vi "On Click Enumerate Cameras.vi"(8 "error in (no error)":errorcluster, 10 "Value":bool, 11 "App in":refnum<class "App.lvclass">) -> (0 "error out":errorcluster, 3 "App out":refnum<class "App.lvclass">)   [LabVIEW 2020, in "AR Example.lvlib" / "App.lvclass"]
uses:
  App.lvclass
  App.lvclass/App.ctl
  b0e96125-61a1-4303-b342-3e2cae2d3e9f.vi
  917a6586-ad63-4fd0-8dd0-0daf31f14cd0.vi
  <vilib>/Comparison/Equal/Equal Functor/Equal Functor.lvclass
  UI/UI.lvclass
  g_ar_toolkit.capture/CameraStream/CameraStream.lvclass
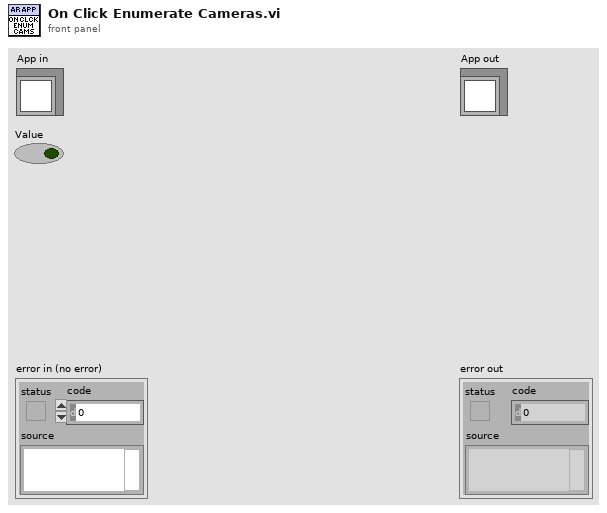
[diagram p1: front panel]
types:
  T1 = enum16{"Set UI Pre Enum", "Enumerate", "Update Lists", "Set UI Post Enum"}
  T2 = enum16{"Set UI Pre Enum", "Enumerate", "Update Lists", "Set UI Post Enum"}[]
  T3 = typedef "g_ar_toolkit.capture.lvlib/CameraStream.lvclass/Device Enumeration.ctl" = cluster{"Name":string, "Streams":set{T4}}
  T4 = typedef "g_ar_toolkit.capture.lvlib/CameraStream.lvclass/Stream Parameters.ctl" = cluster{"Width":u16, "Height":u16, "FPS":u8}
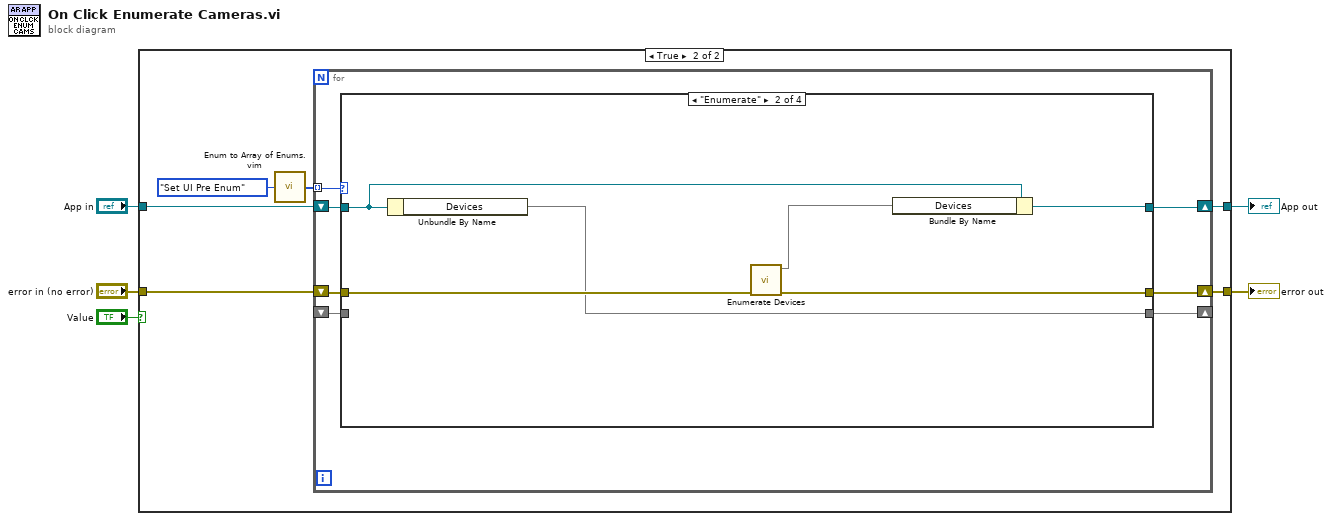
[diagram p0: block diagram]
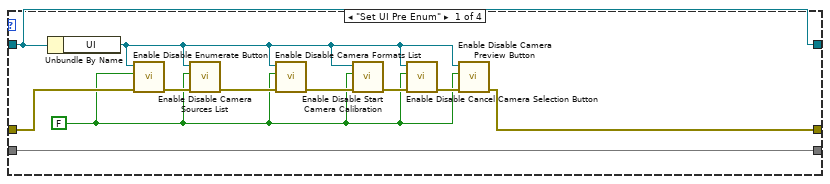
[diagram p3: hidden frame]
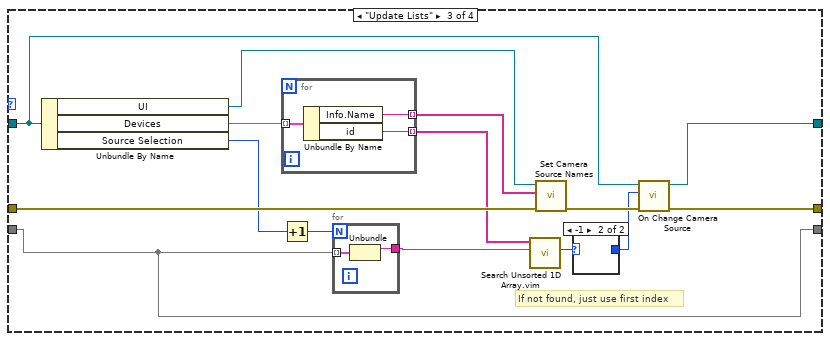
[diagram p4: hidden frame]
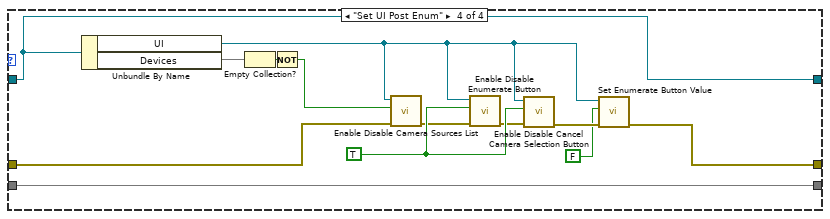
[diagram p6: hidden frame]
diagram:
  n1 = case shown="True" "Value" {
    tunnel: "App in" -> [w6 w13]
    tunnel: "error in (no error)" -> [w7 w12]
    tunnel: [w7 w11] -> w3
    tunnel: [w6 w10] -> w2
    frame False {
    }
    frame True {
      n2 = call "Enum to Array of Enums.vim"("enum"=T1."Set UI Pre Enum") -> ("array of enums"=w8:T2)
      n3 = for {
        shift-right: [w19] -> w11
        shift-left: w12 -> [w20]
        shift-right: [w16] -> w10
        shift-left: w13 -> [w18]
        tunnel: w8 -> [w17] mode=indexing
        shift-right: [w15] -> _
        shift-left: _ -> [w14]
        n4 = case shown="\"Enumerate\"" w17 {
          tunnel: w20 -> [w31 w37 w50 w61]
          tunnel: [w21 w34 w44 w65] -> w19
          tunnel: w18 -> [w26 w36 w46 w70]
          tunnel: [w26 w35 w45 w70] -> w16
          tunnel: [w25 w33 w52 w69] -> w15
          tunnel: w14 -> [w25 _ w52 w69]
          frame "Set UI Pre Enum" {
            w22 = FALSE ("Enable?")
            n5 = Unbundle By Name(w26) -> ("UI"=w23:refnum<class "UI.lvclass">)
            n6 = call-dynamic "Enable Disable Enumerate Button.vi"("error in (no error)"=w31, "Enable?"=w22, "UI in"=w23) -> ("error out"=w30:errorcluster)  [unwired: 8 in]
            n7 = call-dynamic "Enable Disable Camera Sources List.vi"("error in (no error)"=w30, "Enable?"=w22, "UI in"=w23) -> ("error out"=w29:errorcluster)  [unwired: 8 in]
            n8 = call-dynamic "Enable Disable Camera Formats List.vi"("error in (no error)"=w29, "Enable?"=w22, "UI in"=w23) -> ("error out"=w28:errorcluster)  [unwired: 8 in]
            n9 = call-dynamic "Enable Disable Start Camera Calibration.vi"("error in (no error)"=w28, "Enable?"=w22, "UI in"=w23) -> ("error out"=w27:errorcluster)  [unwired: 8 in]
            n10 = call-dynamic "Enable Disable Cancel Camera Selection Button.vi"("error in (no error)"=w27, "Enable?"=w22, "UI in"=w23) -> ("error out"=w24:errorcluster)  [unwired: 8 in]
            n11 = call-dynamic "Enable Disable Camera Preview Button.vi"("error in (no error)"=w24, "Enable?"=w22, "UI in"=w23) -> ("error out"=w21:errorcluster)  [unwired: 8 in]
          }
          frame "Enumerate" {
            n12 = Unbundle By Name(w36) -> ("Devices"=w33:map{string, T3})
            n13 = call "Enumerate Devices.vi"("error in (no error)"=w37) -> ("error out"=w34:errorcluster, "Devices"=w32:map{string, T3})  [unwired: 9 in]
            n14 = Bundle By Name(cluster=w36, "Devices"=w32) -> (w35:refnum<class "App.lvclass">)
          }
          frame "Update Lists" {
            # "If not found, just use first index"
            n15 = Unbundle By Name(w46) -> ("UI"=w49:refnum<class "UI.lvclass">, "Devices"=w51:map{string, T3}, "Source Selection"=w43:i32)
            n16 = for {
              tunnel: w51 -> [w58] mode=indexing
              tunnel: [w57] -> w48 mode=indexing
              tunnel: [w56] -> w42 mode=indexing
              n17 = Unbundle By Name(w58) -> ("Info.Name"=w57:string, "id"=w56:string)
            }
            n18 = Increment(x=w43) -> (x+1=w38:i32)
            n19 = for {
              N: w38 -> [_]
              tunnel: w52 -> [w55] mode=indexing
              tunnel: [w54] -> w41
              n20 = Unbundle(w55) -> ("id"=w54:string)  [unwired: 1 out]
            }
            n21 = call "Search Unsorted 1D Array.vim"("element"=w41, "unsorted 1D array"=w42) -> ("index of element"=w40:i32)  [unwired: 9 in]
            n22 = call-dynamic "Set Camera Source Names.vi"("error in (no error)"=w50, "Names"=w48, "UI in"=w49) -> ("error out"=w47:errorcluster)  [unwired: 8 in]
            n23 = case shown="-1" w40 {
              selector: w40 -> [w53 _]
              tunnel: [w53 _] -> w39
              frame Default {
              }
              frame -1 {
              }
            }
            n24 = call "On Change Camera Source.vi"("error in (no error)"=w47, "Selection"=w39, "App in"=w46) -> ("error out"=w44:errorcluster, "App out"=w45:refnum<class "App.lvclass">)  [unwired: 7 in]
          }
          frame "Set UI Post Enum" {
            w62 = TRUE ("Enable?")
            n25 = Unbundle By Name(w70) -> ("UI"=w64:refnum<class "UI.lvclass">, "Devices"=w68:map{string, T3})
            n26 = Empty Collection?(1:w68) -> (0:w67:bool)
            n27 = Not(x=w67) -> (.not. x?=w66:bool)
            n28 = call-dynamic "Enable Disable Camera Sources List.vi"("error in (no error)"=w61, "Enable?"=w66, "UI in"=w64) -> ("error out"=w60:errorcluster)  [unwired: 8 in]
            n29 = call-dynamic "Enable Disable Enumerate Button.vi"("error in (no error)"=w60, "Enable?"=w62, "UI in"=w64) -> ("error out"=w59:errorcluster)  [unwired: 8 in]
            n30 = call-dynamic "Enable Disable Cancel Camera Selection Button.vi"("error in (no error)"=w59, "Enable?"=w62, "UI in"=w64) -> ("error out"=w71:errorcluster)  [unwired: 8 in]
            n31 = call-dynamic "Set Enumerate Button Value.vi"("error in (no error)"=w71, "Values"=FALSE, "UI in"=w64) -> ("error out"=w65:errorcluster)  [unwired: 8 in]
          }
        }
      }
    }
  }
  "error out" <- w3
  "App out" <- w2
